vi "DDE Master Control.vi"(5 "timeout(-1)":i32=-1, 9 "input":T2={"trans type"=1, "refnums"=[], "data1"="excel", "data2"="sheet1", "status"=FALSE} {"refnums" format="%.0x"}) -> (0 "error out":errorcluster, 1 "changed?":bool, 2 "data":string, 3 "refnum":u32 format="%.0x", 4 "changed values":T1(array[cluster]))   [LabVIEW 2018]
panel:
  in  "datatype":T1(array[cluster])
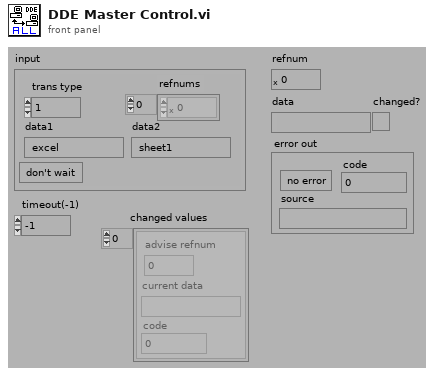
[diagram p1: front panel]
types:
  T1 = cluster{"advise refnum":u32, "current data":string, "code":i32}[]
  T2 = cluster{"trans type":i8, "refnums":u32[], "data1":string, "data2":string, "status":bool}
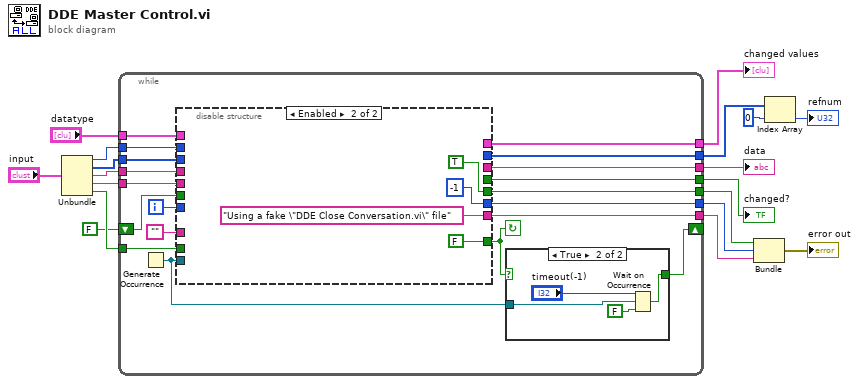
[diagram p0: block diagram]
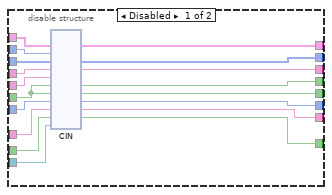
[diagram p2: hidden frame]
diagram:
  n1 = Unbundle("input") -> ("trans type"=w12:i8, "refnums"=w9:u32[], "data1"=w17:string, "data2"=w15:string, "status"=w8:bool)
  n2 = while {
    tunnel: "datatype" -> [w19]
    tunnel: [w20] -> w2
    tunnel: [w22] -> w6
    shift-left: FALSE -> [w21]
    shift-right: [w24] -> _
    tunnel: w8 -> [w25]
    tunnel: [w27] -> w4
    tunnel: w9 -> [w28]
    tunnel: [w34] -> w14
    tunnel: [w35] -> w13
    tunnel: w15 -> [w31]
    tunnel: w17 -> [w36]
    tunnel: [w33] -> w16
    tunnel: [w37] -> w10
    tunnel: w12 -> [w30]
    i -> [w23]
    stop <- w26 continue-if-true
    n3 = Generate Occurrence() -> (w29:refnum<k4>)
    n4 = disable-structure shown="Enabled" {
      disable-tunnel: [w55 "Using a fake \"DDE Close Conversation.vi\" file" ("source")] -> w37
      disable-tunnel: w36 -> [w54 _]
      disable-tunnel: [w53 _] -> w35
      disable-tunnel: [w52 TRUE ("status")] -> w34
      disable-tunnel: [w51 -1 ("code")] -> w33
      disable-tunnel: "" -> [w50 _]
      disable-tunnel: w31 -> [w49 _]
      disable-tunnel: w30 -> [w48 _]
      disable-tunnel: w29 -> [w47 _]
      disable-tunnel: w28 -> [w46 _]
      disable-tunnel: [w45 _] -> w27
      disable-tunnel: [w44 FALSE ("status")] -> w26
      disable-tunnel: w25 -> [w43 _]
      disable-tunnel: w23 -> [w42 _]
      disable-tunnel: [w41 _] -> w22
      disable-tunnel: w21 -> [w40 _]
      disable-tunnel: [w39 _] -> w20
      disable-tunnel: w19 -> [w38 _]
      frame Disabled {
        n5 = cin(w38, w48, w46, w54, w49, w40, w40, w42, w50, w43, w47) -> (w39:T1, w45:u32[], w53:string, w41:bool, w52:bool, w51:i32, w55:string, w44:bool)  [unwired: 3 in]
      }
      frame Enabled {
      }
    }
    n6 = case shown="True" w26 {
      selector: w26 -> [w60 _]
      tunnel: w29 -> [_ w64]
      tunnel: [w60 w61] -> w24
      frame False {
      }
      frame True {
        n7 = Wait on Occurrence(1:FALSE, 2:w64, 3:"timeout(-1)") -> (0:w61:bool)
      }
    }
  }
  "data" <- w13
  "changed?" <- w6
  "changed values" <- w2
  n8 = Bundle("status"=w14, "code"=w16, "source"=w10) -> (→"error out":errorcluster)  [unwired: 1 in]
  n9 = Index Array(array=w4, index=0) -> (element=→"refnum":u32)
